vi "Mixture_similarity_map_data.vi"(10 "Mixture components":T1(array[cluster]), 11 "Odour component data":T2) -> (3 "input cluster":cluster{"MDS1":dbl[], "MDS2":dbl[]})   [LabVIEW 2016]
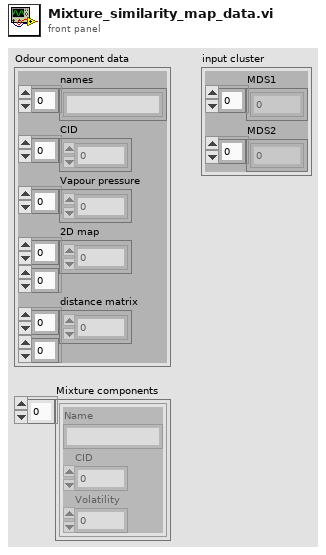
[diagram p1: front panel]
types:
  T1 = cluster{"Name":string, "CID":i32, "Volatility":dbl}[]
  T2 = cluster{"names":string[], "CID":i32[], "Vapour pressure":dbl[], "2D map":dbl[][], "distance matrix":dbl[][]}
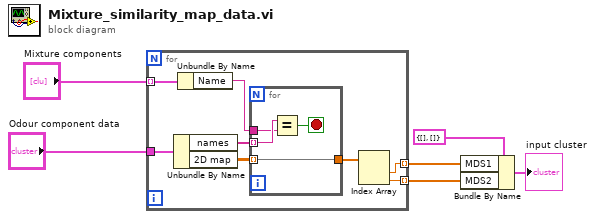
[diagram p0: block diagram]
diagram:
  n1 = for {
    tunnel: "Mixture components" -> [w14] mode=indexing
    tunnel: "Odour component data" -> [w13]
    tunnel: [w9] -> w3 mode=indexing
    tunnel: [w8] -> w4 mode=indexing
    n2 = Unbundle By Name(w13) -> ("names"=w12:string[], "2D map"=w7:dbl[][])
    n3 = Unbundle By Name(w14) -> ("Name"=w11:string)
    n4 = for {
      tunnel: w12 -> [w18] mode=indexing
      tunnel: w11 -> [w17]
      tunnel: w7 -> [w16] mode=indexing
      tunnel: [w16] -> w10
      stop <- w15 stop-if-true
      n5 = Equal?(x=w18, y=w17) -> (x = y?=w15:bool)
    }
    n6 = Index Array(array=w10) -> (element #1=w9:dbl, element #2=w8:dbl)  [unwired: 2 in]
  }
  n7 = Bundle By Name(cluster=cluster{"MDS1":dbl[], "MDS2":dbl[]} {"MDS1"=[], "MDS2"=[]} ("input cluster"), "MDS1"=w3, "MDS2"=w4) -> (→"input cluster":cluster{"MDS1":dbl[], "MDS2":dbl[]})
